vi "stepper contorl simulation.vi"() -> ()   [LabVIEW 2017]
panel:
  out "appended array":bool[](array[boolean])
  out "Motor Controll Voltage":dynamicdata(graph)
  in  "Run":bool
  out "Delaty time":i32
  in  "Speed":i32(slide) scale=0.0..20.0
  out "At stepp":i32
  in  "Direction":bool
  in  "Halfstepp":bool
  in  "Quit":bool
  out "P3":bool
  out "P2":bool
  out "P1":bool
  out "P0":bool
  in  "Motor controll enable":bool
  in  "Steps":i32
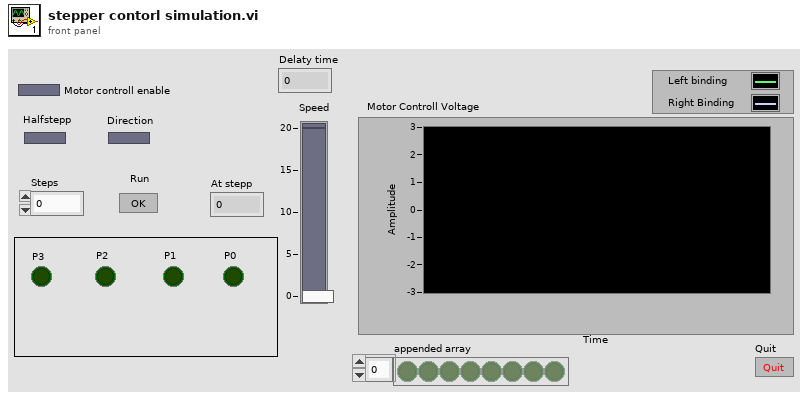
[diagram p1: front panel]
types:
  T1 = cluster{"Boolean 4":bool, "Boolean 3":bool, "Boolean 2":bool, "Boolean":bool}
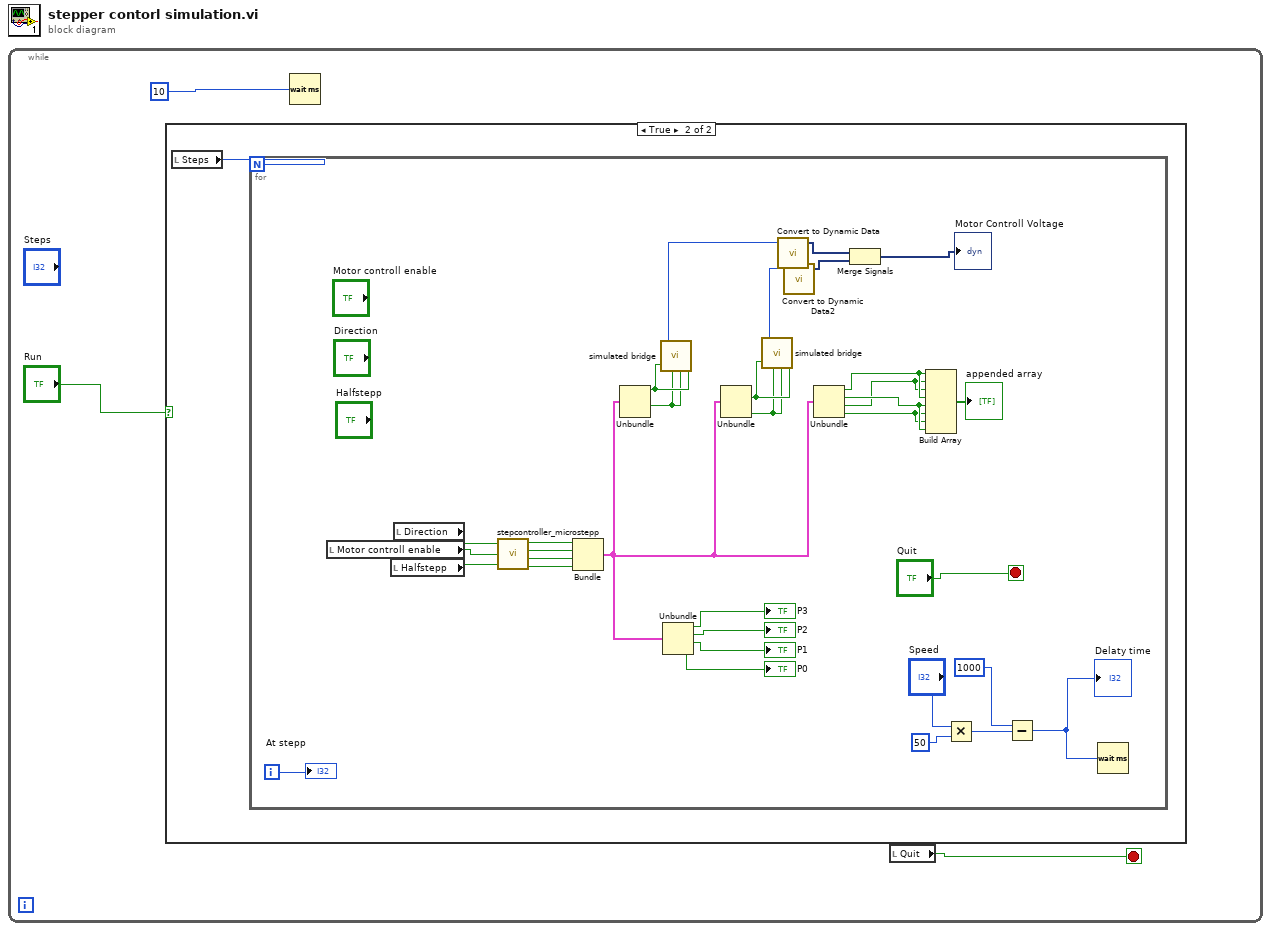
[diagram p0: block diagram]
diagram:
  n1 = while {
    stop <- w3 stop-if-true
    n2 = case shown="True" "Run" {
      frame False {
      }
      frame True {
        n3 = local read "Steps"() -> (w4:i32)
        n4 = for {
          N: w4 -> [_]
          i -> [w37]
          stop <- "Quit" stop-if-true
          n5 = local read "Motor controll enable"() -> (w35:bool)
          n6 = local read "Halfstepp"() -> (w34:bool)
          n7 = local read "Direction"() -> (w36:bool)
          n8 = call "stepcontroller_microstepp.vi"("microstep"=w34, "motor stopp"=w35, "Direction"=w36) -> ("Boolean"=w25:bool, "Boolean 2"=w26:bool, "Boolean 3"=w27:bool, "Boolean 4"=w28:bool)  [unwired: 1 in]
          n9 = Bundle("Boolean 4"=w28, "Boolean 3"=w27, "Boolean 2"=w26, "Boolean"=w25) -> (w24:T1)  [unwired: 1 in]
          n10 = Unbundle(w24) -> ("Boolean 4"=w18:bool, "Boolean 2"=w16:bool)  [unwired: 2 out]
          n11 = call "simulated bridge.vi"("s4"=w18, "s3"=w16, "s2"=w16, "s1"=w18) -> ("Motor voltage"=w33:i8)  [unwired: 1 out]
          n12 = Unbundle(w24) -> ("Boolean 4"=→"P3":bool, "Boolean 3"=→"P2":bool, "Boolean 2"=→"P1":bool, "Boolean"=→"P0":bool)
          n13 = Unbundle(w24) -> ("Boolean 3"=w17:bool, "Boolean"=w15:bool)  [unwired: 2 out]
          n14 = call "simulated bridge.vi"("s4"=w17, "s3"=w15, "s2"=w15, "s1"=w17) -> ("Motor voltage"=w32:i8)  [unwired: 1 out]
          n15 = call "Convert to Dynamic Data"("Double"=w33) -> ("Dynamic Data Type"=w29:dynamicdata)  [unwired: 3 in]
          n16 = call "Convert to Dynamic Data2"("Double"=w32) -> ("Dynamic Data Type"=w30:dynamicdata)  [unwired: 3 in]
          n17 = Unbundle(w24) -> ("Boolean 4"=w14:bool, "Boolean 3"=w13:bool, "Boolean 2"=w12:bool, "Boolean"=w11:bool)
          n18 = Merge Signals(w29, w30) -> (→"Motor Controll Voltage":dynamicdata)
          n19 = Build Array(w14, w12, w12, w14, w13, w11, w11, w13) -> (→"appended array":bool[])
          n20 = Multiply(x="Speed", y=50) -> (x*y=w10:i32)
          n21 = Subtract(x=1000 ("y"), y=w10) -> (x-y=w5:i32)
          "Delaty time" <- w5
          n22 = Wait (ms)(milliseconds to wait=w5) -> ()  [unwired: 1 out]
          "At stepp" <- w37
        }
      }
    }
    n23 = Wait (ms)(milliseconds to wait=u32 10) -> ()  [unwired: 1 out]
    n24 = local read "Quit"() -> (w3:bool)
  }
